vi "fpga_Resampling (M Class_50Hz).vi"(0 "signal in":fxp<+/-,24,1>, 1 "number of channels":T2=7 items=["1"=1, "2"=2, "3"=3, "4"=4, "5"=5, "6"=6, "7"=7, "8"=8, "9"=9, "10"=10, "11"=11, "12"=12, "13"=13, "14"=14, "15"=15, "16"=16], 2 "Memory In":refnum<k21>, 5 "timestamp [s]":fxp<+,64,32> format="%.42g", 7 "reference channel index":u8, 9 "input data valid? (T)":bool=TRUE, 12 "ready for output? (T)":bool=TRUE) -> (4 "resampled data":T1, 10 "output valid":bool, 14 "ready for input":bool, 15 "error":i32)   [LabVIEW 2013, in "NI_EP_PMU_FPGA.lvlib"]
doc: "Converts even-time-spaced voltage and current signals to even-angle-spaced signals by resampling the voltage and current signals using a sampling rate of 50 kHz. The output signals are synchronous to the line frequency with a constant number of samples per cycle."
uses:
  <vilib>/addons/Electrical Power/PMU/NI_EP_PMU_FPGA.lvlib
  <vilib>/addons/Electrical Power/PQ/Resampling/FPGA/subVIs/fpga_NofCH.ctl
  <vilib>/addons/Electrical Power/PQ/Resampling/FPGA/subVIs/fpga_Resampled.ctl
  <vilib>/addons/Electrical Power/PQ/Resampling/FPGA/subVIs/fpga_Typedef Fnom.ctl
  <vilib>/addons/Electrical Power/PQ/Resampling/NI_EP_Resample_FPGA.lvlib
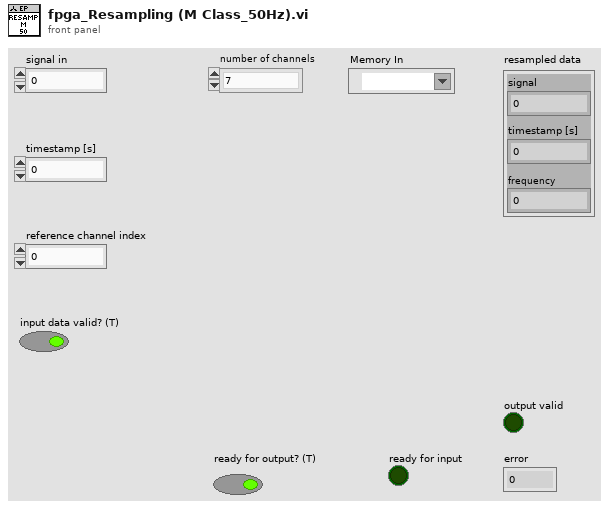
[diagram p1: front panel]
types:
  T1 = typedef "NI_EP_Resample_FPGA.lvlib/fpga_Resampled.ctl" = cluster{"signal":fxp<+/-,32,3>, "timestamp [s]":fxp<+,64,32>, "frequency":fxp<+,32,8>}
  T2 = typedef "NI_EP_Resample_FPGA.lvlib/fpga_NofCH.ctl" = u8
  T3 = typedef "NI_EP_Resample_FPGA.lvlib/fpga_Typedef Fnom.ctl" = u8
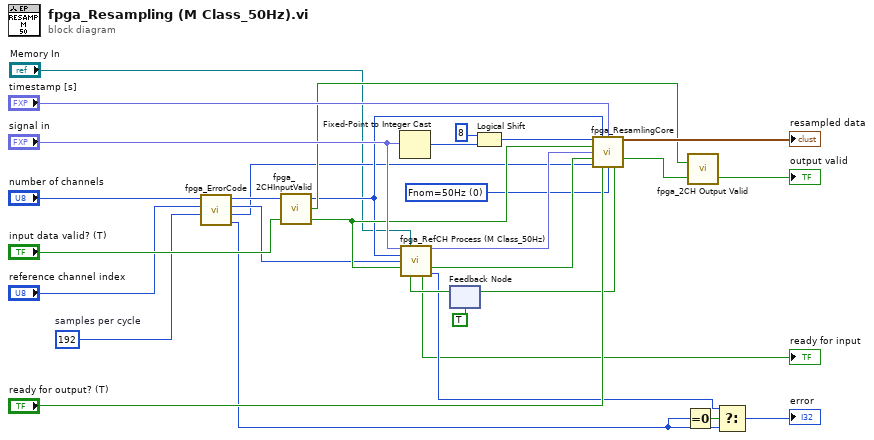
[diagram p0: block diagram]
diagram:
  w7 = u16 192  # samples per cycle
  w8 = T3 0 items=["Fnom=50Hz", "Fnom=60Hz"] ("Fnom")
  n1 = call <vilib>:"fpga_ErrorCode.vi"("samples per cycle"=w7, "reference channel index"="reference channel index", "number of channels"="number of channels") -> ("error"=w3:i32, "samples per cycle out"=w9:u16, "ref channel index out"=w10:u8, "number of CH out"=w11:u8)  [unwired: 5 in]
  n2 = call <vilib>:"fpga_2CHInputValid.vi"("input data valid"="input data valid? (T)", "Channel number"=w11) -> ("input valid"=w19:bool, "1CH?"=w21:bool, "Channel number"=w12:u8)  [unwired: 1 in]
  n3 = Fixed-Point to Integer Cast(1:"signal in") -> (0:w14:i32)
  n4 = feedback #1(TRUE ("Ready for reference input")) -> (w18:bool)
  n5 = call <vilib>:"fpga_RefCH Process (M Class_50Hz).vi"("data in <?24.1>"="signal in", "Memory In"="Memory In", "Channel number"=w12, "Reference index"=w10, "input data valid"=w19, "ready for output"=w18) -> ("Filtered Ref data"=w17:fxp<+/-,24,3>, "output valid"=w16:bool, "ready for input"=→"ready for input":bool, "error"=w2:i32)  [unwired: 6 in]
  n6 = Logical Shift(y=i8 8, x=w14) -> (x << y=w13:i32)
  n7 = call <vilib>:"fpga_ResamlingCore.vi"("data in"=w13, "Channel number"=w12, "timestamp"="timestamp [s]", "input data valid"=w19, "reference in"=w17, "input reference valid"=w16, "interpolation factor"=w9, "Ready for output"="ready for output? (T)", "Fnom"=w8) -> ("Resample data and time"=→"resampled data":T1, "output valid"=w20:bool, "Ready for reference input"=w23:bool)  [unwired: 2 in, 2 out]
  n8 = feedback-in #1(w23) -> ()
  n9 = Equal To 0?(x=w3) -> (x = 0?=w5:bool)
  n10 = call <vilib>:"fpga_2CH Output Valid.vi"("output valid"=w20, "1CH?"=w21) -> ("output valid"=→"output valid":bool)  [unwired: 1 in]
  n11 = Select(t=w2, s=w5, f=w3) -> (s? t:f=→"error":i32)
